vi "Lesson Launcher.vi"() -> ()   [LabVIEW 2020]
panel:
  out "error out":errorcluster
  out "error out Process":errorcluster
  out "error out AQN":errorcluster
  in  "error in":errorcluster
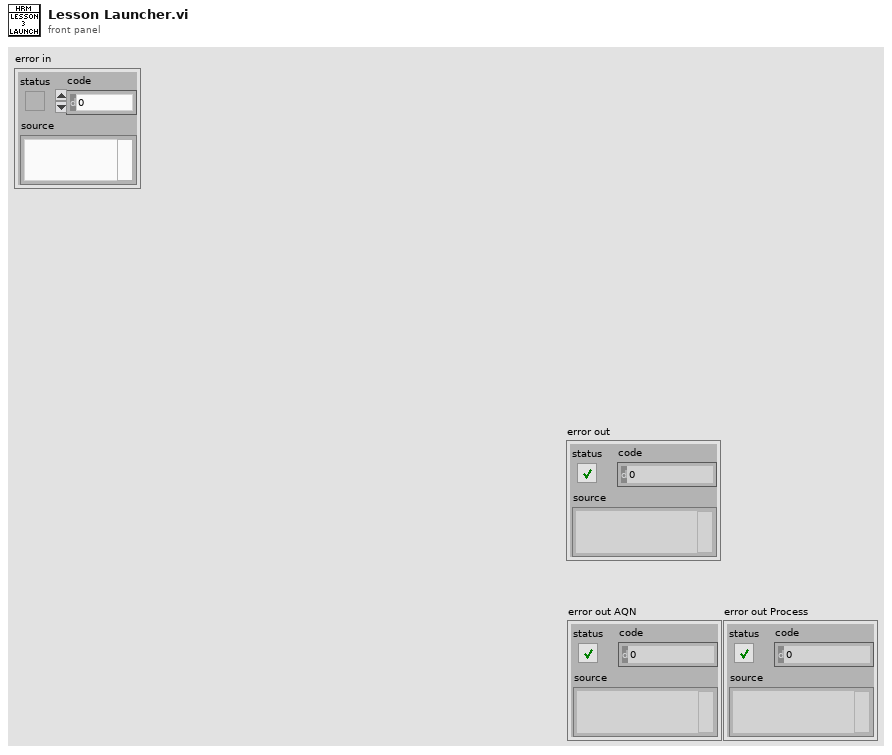
[diagram p1: front panel]
types:
  T1 = typedef "HRM-init-cluster.ctl" = cluster{"User Events":T2, "Intial State":T3}
  T2 = typedef "HRM-init-user_events.ctl" = cluster{"Additional Signal to remove [s]":refnum<user-event>, "samples [s]":refnum<user-event>, "Heart Rate":refnum<user-event>, "Raw collected data":refnum<user-event>, "Filtered data":refnum<user-event>, "Raw Data":refnum<user-event>, "stop":refnum<user-event>, "Status Feedback":refnum<user-event>, "pause AQN":refnum<user-event>, "Clear wf Data":refnum<user-event>, "Pulse settings":refnum<user-event>}
  T3 = typedef "HRM-init-Intial State.ctl" = cluster{"Pause AQN":bool, "Hardware type":T4, "Pulse settings":T5}
  T4 = typedef "HRM-init-hardware_selector.ctl" = enum16{"Simulator", "myDAQ", "Arduino", "Analog Discovery"}
  T5 = typedef "HRM-process-Pulse settings.ctl" = cluster{"Manual?":bool, "Top":dbl, "Bottom":dbl}
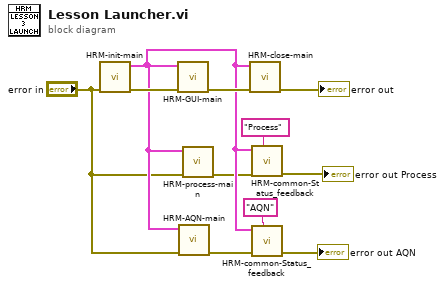
[diagram p0: block diagram]
diagram:
  n1 = call "HRM-init-main.vi"("error in (no error)"="error in") -> ("error out"=w11:errorcluster, "init cluster"=w6:T1)  [unwired: 9 in]
  n2 = call "HRM-GUI-main.vi"("error in (no error)"=w11, "init cluster"=w6) -> ("error out"=w9:errorcluster)  [unwired: 9 in]
  n3 = call "HRM-AQN-main.vi"("error in (no error)"="error in", "init cluster"=w6) -> ("error out"=w7:errorcluster)  [unwired: 9 in]
  n4 = call "HRM-process-main.vi"("error in (no error)"="error in", "init cluster"=w6) -> ("error out"=w3:errorcluster)  [unwired: 9 in]
  n5 = call "HRM-close-main.vi"("error in (no error)"=w9, "init cluster"=w6) -> ("error out"=→"error out":errorcluster)  [unwired: 9 in]
  n6 = call "HRM-common-Status_feedback.vi"("Module name"="Process", "error in (no error)"=w3, "init cluster"=w6) -> ("error out"=→"error out Process":errorcluster)  [unwired: 8 in]
  n7 = call "HRM-common-Status_feedback.vi"("Module name"="AQN", "error in (no error)"=w7, "init cluster"=w6) -> ("error out"=→"error out AQN":errorcluster)  [unwired: 8 in]
